vi "Send Email to Multiple.vi"(9 "Message":string, 10 "Subject":string, 11 "To:":string[](array[string])=["sfricke@chromaus.com", "cobrasysin@chromaus.com"]) -> ()   [LabVIEW 2019, in "GUI.lvlib"]
uses:
  GUI.lvlib
panel:
  in  "error in (no error)":errorcluster
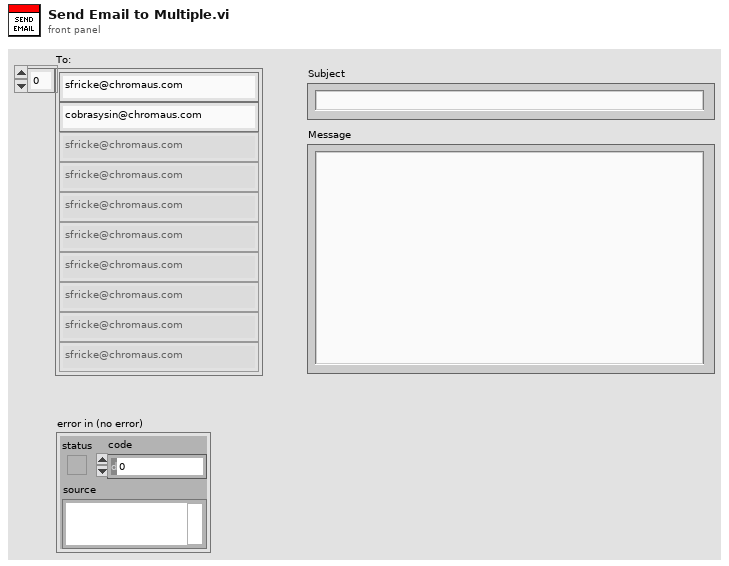
[diagram p1: front panel]
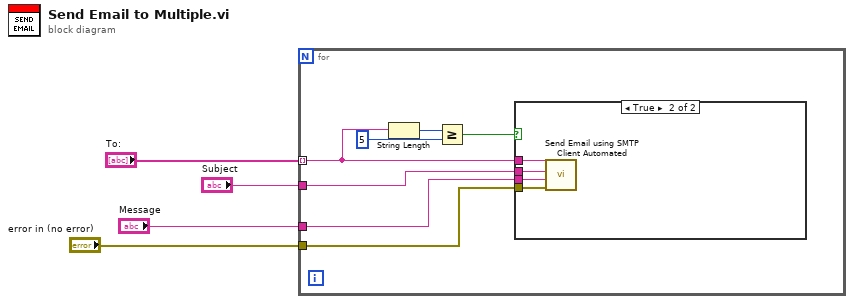
[diagram p0: block diagram]
diagram:
  n1 = for {
    tunnel: "To:" -> [w8] mode=indexing
    tunnel: "error in (no error)" -> [w11]
    tunnel: "Subject" -> [w10]
    tunnel: "Message" -> [w9]
    n2 = String Length(string=w8) -> (length=w7:i32)
    n3 = Greater Or Equal?(x=w7, y=5) -> (x >= y?=w5:bool)
    n4 = case shown="True" w5 {
      tunnel: w11 -> [_ w15]
      tunnel: w10 -> [_ w14]
      tunnel: w9 -> [_ w13]
      tunnel: w8 -> [_ w12]
      frame False {
      }
      frame True {
        n5 = call "Send Email using SMTP Client Automated.vi"("error in (no error)"=w15, "Message"=w13, "Subject"=w14, "To:"=w12) -> ()  [unwired: 8 in]
      }
    }
  }
